vi "Begin.vi"(8 "error in":errorcluster) -> (0 "error out":errorcluster)   [LabVIEW 2017]
doc: "Called before other user functions, this VI can be used to open I/O refnums, load in file data, and do general program initialization. Notice that the <B>error out</B> terminal is simply used for data flow. Wiring it to other structures or subVIs ensures that this VI runs first."
uses:
  <vilib>/Rock Robotics/WPI/DriverStation/WPI_DriverStationRobotMode2.ctl
  <vilib>/Rock Robotics/WPI/Joystick/WPI_JoystickDeviceEnum.ctl
  <vilib>/Rock Robotics/SystemInterfaces/spilib/spi_bus.ctl
  Robot Global Data.vi
  <vilib>/Rock Robotics/Network Tables/NT Write String Array.vi
  <vilib>/Rock Robotics/Network Tables/NT Write Boolean.vi
  <vilib>/Rock Robotics/WPI/Gyro/WPI_GyroXRS450_SPI_Open.vi
  <vilib>/Rock Robotics/Network Tables/NT Read Number.vi
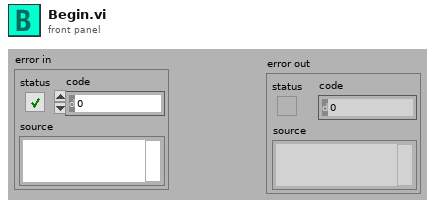
[diagram p1: front panel]
types:
  T1 = typedef "WPI_JoystickDeviceEnum.ctl" = enum16{"USB 0", "USB 1", "USB 2", "USB 3", "USB 4", "USB 5"}
  T2 = typedef "spi_bus.ctl" = enum16{"SPI On-Board, CS0", "SPI On-Board, CS1", "SPI On-Board, CS2", "SPI On-Board, CS3", "SPI MXP", "Invalid"}
  T3 = typedef "WPI_DriverStationRobotMode2.ctl" = enum16{"Autonomous Disabled", "Autonomous Enabled", "Teleop Disabled", "Teleop Enabled", "Disconnected", "Finish", "Test Disabled", "Test Enabled", "Emergency Stopped"}
  T4 = typedef "WPI_JoystickDevRef.ctl" = cluster{"Device":T1}
  T5 = typedef "WPI_GyroDevRef.ctl" = cluster{"DevStatus":errorcluster, "Analog Channel":T6, "Gain (VoltsPerDegree/Second)":dbl, "Gyro Type":enum16{"Analog", "XRS450"}, "Handle":i32, "SPI Bus":T2, "Device Found":bool, "Sample Rate":dbl, "Calibrate On Open":bool, "Offset":dbl}
  T6 = typedef "FPGA_AIChannel.ctl" = enum8{"AI 0", "AI 1", "AI 2", "AI 3", "AI MXP 0", "AI MXP 1", "AI MXP 2", "AI MXP 3", "Invalid"}
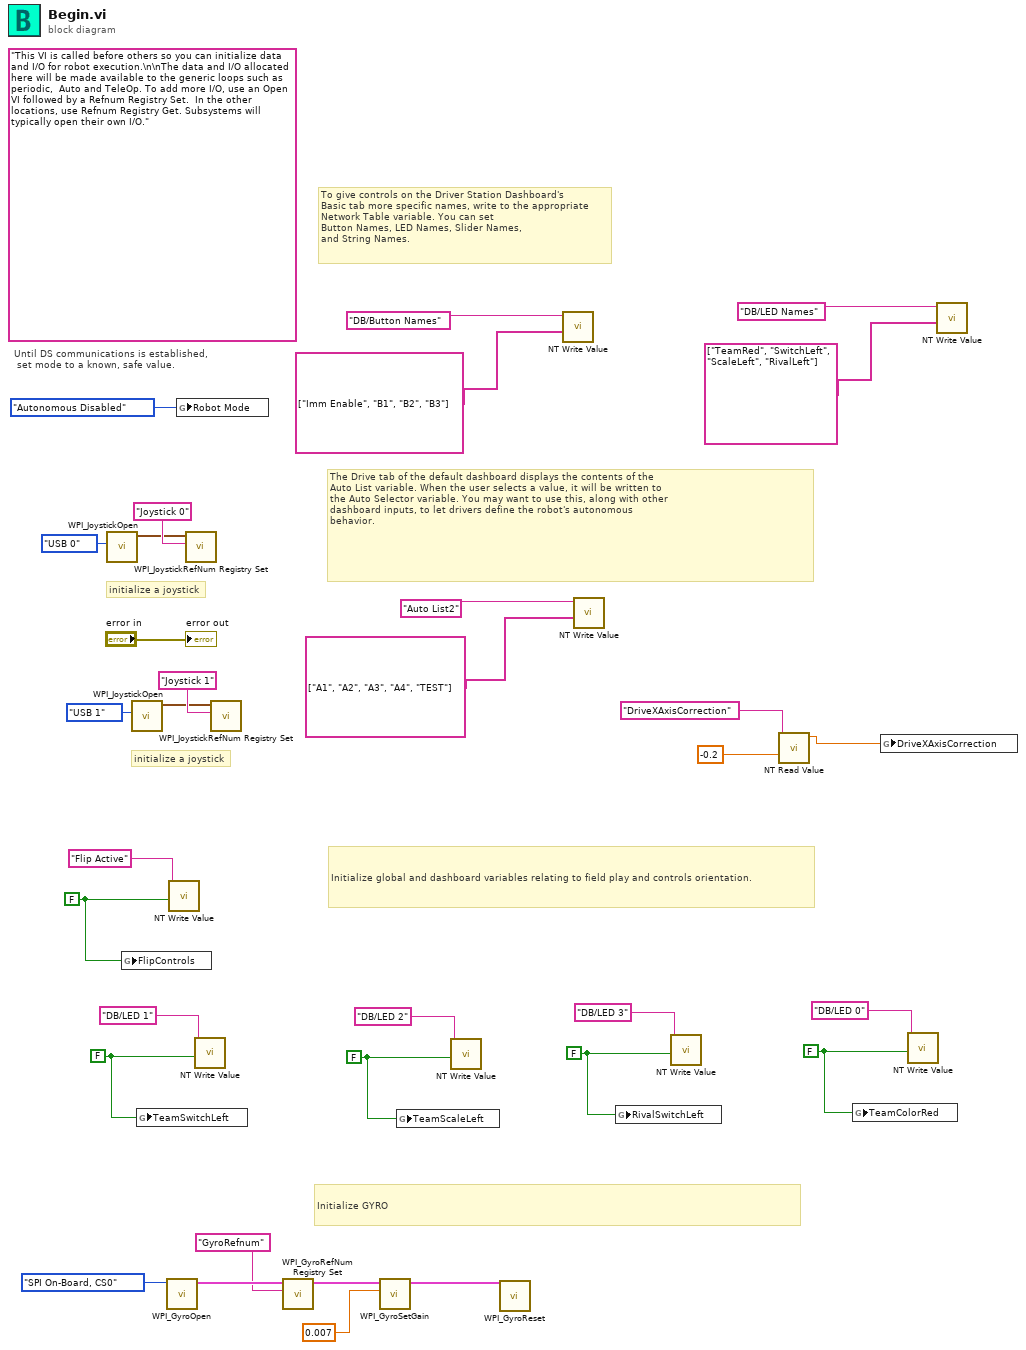
[diagram p0: block diagram]
diagram:
  w15 = FALSE ("Boolean")
  w17 = FALSE ("Boolean")
  w19 = FALSE ("Boolean")
  w21 = FALSE ("Boolean")
  w23 = FALSE ("Boolean")
  (unwired) "This VI is called before others so you can initialize data and I/O for robot execution.\n\nThe data and I/O allocated here will be made available to the generic loops such as periodic,  Auto and TeleOp. To add more I/O, use an Open VI followed by a Refnum Registry Set.  In the other locations, use Refnum Registry Get. Subsystems will typically open their own I/O."
  # "initialize a joystick"
  # "Initialize GYRO"
  # "Initialize global and dashboard variables relating to field play and controls orientation."
  # "The Drive tab of the default dashboard displays the contents of the\nAuto List variable. When the user selects a value, it will be written to\nthe Auto Selector variable. You may want to use this, along with other\ndashboard inputs, to let drivers define the robot's autonomous\nbehavior."
  # "To give controls on the Driver Station Dashboard's\nBasic tab more specific names, write to the appropriate\nNetwork Table variable. You can set\nButton Names, LED Names, Slider Names,\nand String Names."
  # "initialize a joystick"
  # "Until DS communications is established,\n set mode to a known, safe value."
  n1 = call <vilib>:"WPI_JoystickOpen.vi"("JoystickDevice"=WPI_JoystickDeviceEnum."USB 0") -> ("JoystickDevRef"=w31:T4)  [unwired: 10 in]
  n2 = global write "Robot Global Data.vi" "FlipControls"(w23) -> ()
  n3 = call <vilib>:"WPI_JoystickOpen.vi"("JoystickDevice"=WPI_JoystickDeviceEnum."USB 1") -> ("JoystickDevRef"=w5:T4)  [unwired: 10 in]
  n4 = global write "Robot Global Data.vi" "TeamSwitchLeft"(w21) -> ()
  n5 = call-poly <vilib>:"WPI_GyroOpen.vi"("SPI Bus"=spi_bus."SPI On-Board, CS0") -> ("GyroDevRef"=w11:T5)  [unwired: 8 in, 2 out]
  n6 = call-poly <vilib>:"NT Write Value.vi"("Boolean"=w23, "Name"="Flip Active") -> ()  [unwired: 9 in, 1 out]
  n7 = global write "Robot Global Data.vi" "Robot Mode"(WPI_DriverStationRobotMode2."Autonomous Disabled" ("Robot Mode")) -> ()
  n8 = call <vilib>:"WPI_JoystickRefNum Registry Set.vi"("refnum name"="Joystick 0", "JoystickDevRef"=w31) -> ()  [unwired: 8 in, 2 out]
  n9 = call-poly <vilib>:"NT Write Value.vi"("Boolean"=w21, "Name"="DB/LED 1") -> ()  [unwired: 9 in, 1 out]
  n10 = call <vilib>:"WPI_JoystickRefNum Registry Set.vi"("refnum name"="Joystick 1", "JoystickDevRef"=w5) -> ()  [unwired: 8 in, 2 out]
  n11 = call <vilib>:"WPI_GyroRefNum Registry Set.vi"("refnum name"="GyroRefnum", "GyroDevRef"=w11) -> ("GyroDevRef"=w10:T5)  [unwired: 8 in, 1 out]
  n12 = call <vilib>:"WPI_GyroSetGain.vi"("Gain (VoltsPerDegree/Second)"=0.007, "GyroDevRef"=w10) -> ("GyroDevRef"=w7:T5)  [unwired: 8 in, 1 out]
  n13 = global write "Robot Global Data.vi" "TeamScaleLeft"(w19) -> ()
  n14 = call-poly <vilib>:"NT Write Value.vi"("Boolean"=w19, "Name"="DB/LED 2") -> ()  [unwired: 9 in, 1 out]
  n15 = call <vilib>:"WPI_GyroReset.vi"("GyroDevRef"=w7) -> ()  [unwired: 9 in, 2 out]
  n16 = call-poly <vilib>:"NT Write Value.vi"("String Array"=string[] ["Imm Enable", "B1", "B2", "B3"], "Name"="DB/Button Names") -> ()  [unwired: 9 in, 1 out]
  n17 = call-poly <vilib>:"NT Write Value.vi"("String Array"=string[] ["A1", "A2", "A3", "A4", "TEST"], "Name"="Auto List2") -> ()  [unwired: 9 in, 1 out]
  n18 = global write "Robot Global Data.vi" "RivalSwitchLeft"(w17) -> ()
  n19 = call-poly <vilib>:"NT Write Value.vi"("Boolean"=w17, "Name"="DB/LED 3") -> ()  [unwired: 9 in, 1 out]
  n20 = call-poly <vilib>:"NT Read Value.vi"("Default Value"=-0.2, "Name"="DriveXAxisCorrection") -> ("Numeric"=w2:dbl)  [unwired: 8 in, 1 out]
  n21 = global write "Robot Global Data.vi" "TeamColorRed"(w15) -> ()
  n22 = global write "Robot Global Data.vi" "DriveXAxisCorrection"(w2) -> ()
  n23 = call-poly <vilib>:"NT Write Value.vi"("Boolean"=w15, "Name"="DB/LED 0") -> ()  [unwired: 9 in, 1 out]
  n24 = call-poly <vilib>:"NT Write Value.vi"("String Array"=string[] ["TeamRed", "SwitchLeft", "ScaleLeft", "RivalLeft"], "Name"="DB/LED Names") -> ()  [unwired: 9 in, 1 out]
  "error out" <- "error in"
